vi "main--pop up example.vi"() -> ()   [LabVIEW 2021]
doc: "Example for showing different pop-up types"
uses:
  Graphics.ctl
  Popup/message info--typedef.ctl
  Standard/Two Button/Two Button.lvclass
  Pop-Up.lvlib
  Theme/Theme.lvclass
  Standard/Timeout/Timeout.lvclass
  Standard/One Button/One Button.lvclass
  Standard/Input (DBL)/Input (DBL).lvclass
  Custom/Custom - One Button/Custom - One Button.lvclass
  Popup/Popup.lvclass
  user32.dll
panel:
  in  "close":bool
  out "header":bool caption="Boolean"
  out "Value":dbl
  in  "time (seconds)":dbl=2.0
  out "Choice":bool
  in  "two-button":bool
  in  "timeout":bool
  in  "custom":bool
  in  "one-button":bool
  in  "load":bool
  in  "input-dbl":bool
  # "Run this VI to see calling a few different types of Pop-Ups\n->Uses Standard Images for most (change on block diagram to see other options)"
  # "temporarily applies a new \ntheme"
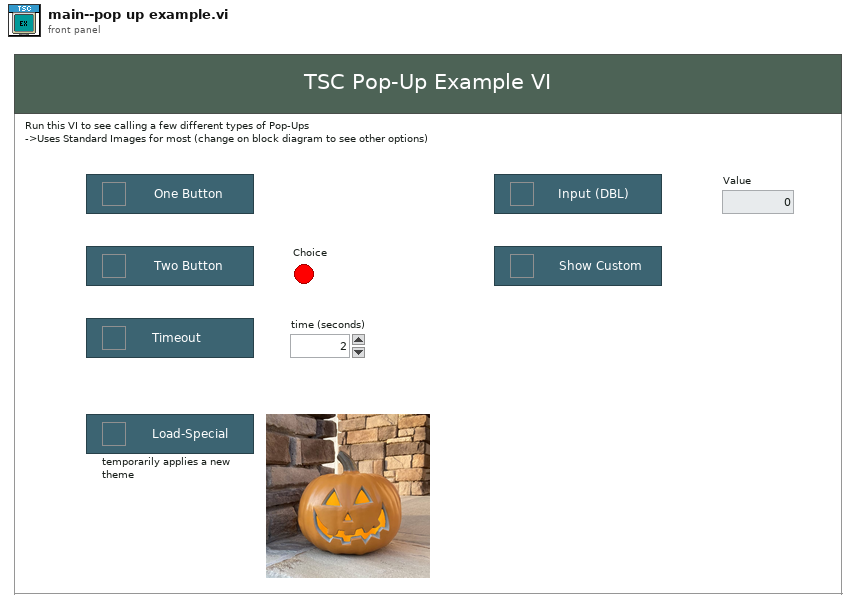
[diagram p1: front panel]
types:
  T1 = typedef "Pop-Up.lvlib/Graphics.ctl" = string
  T2 = typedef "Pop-Up.lvlib/Popup.lvclass/message info--typedef.ctl" = cluster{"Message Height":i32, "Message Width":i32, "Message Location":enum16{"Top", "Bottom", "Right", "Left"}}
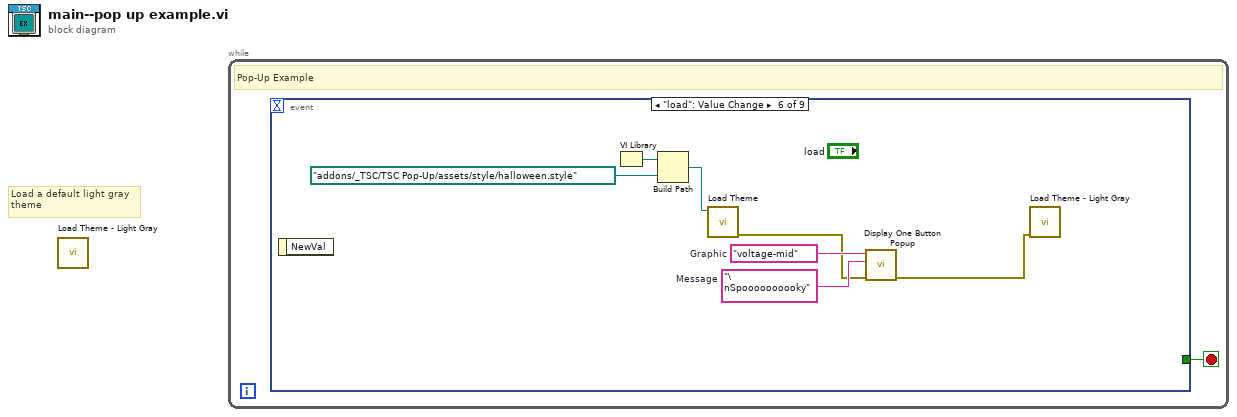
[diagram p0: block diagram]
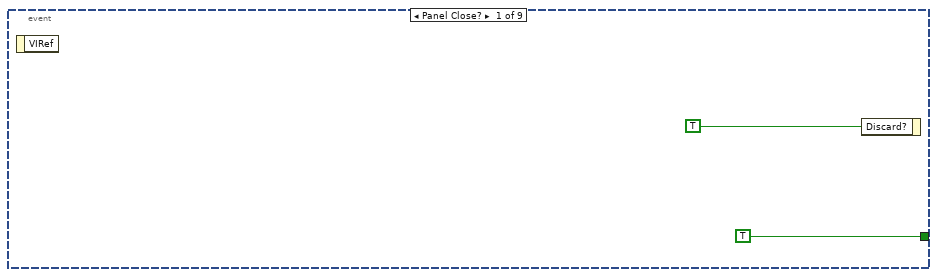
[diagram p2: hidden frame]
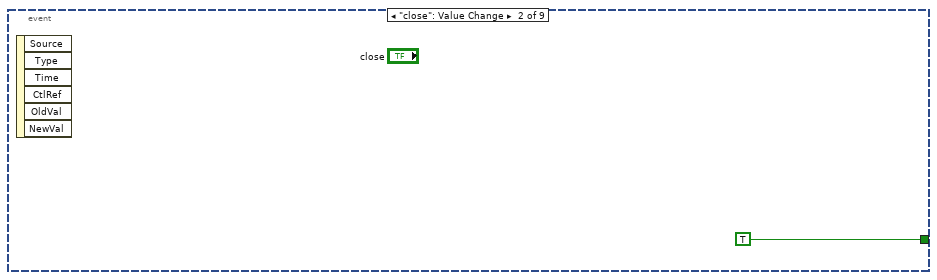
[diagram p3: hidden frame]
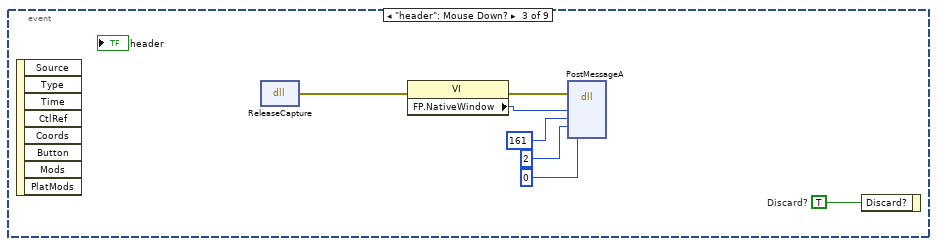
[diagram p4: hidden frame]
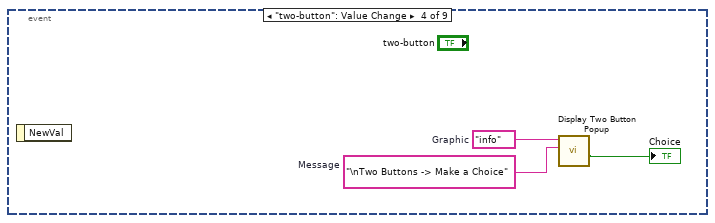
[diagram p5: hidden frame]
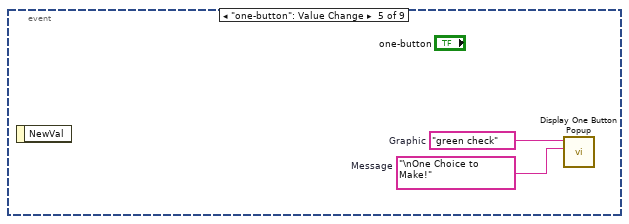
[diagram p6: hidden frame]
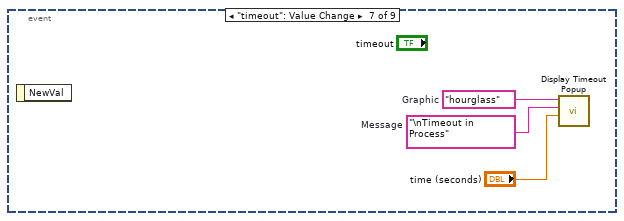
[diagram p7: hidden frame]
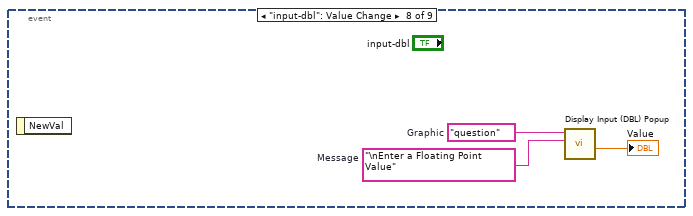
[diagram p8: hidden frame]
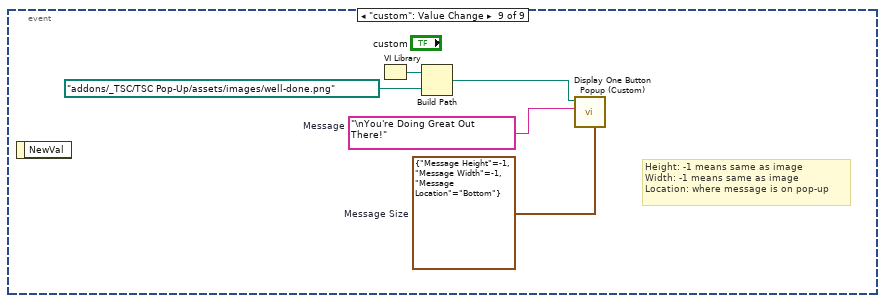
[diagram p9: hidden frame]
diagram:
  # "Load a default light gray\ntheme"
  n1 = call "Load Theme - Light Gray.vi"() -> ()  [unwired: 10 in, 2 out]
  n2 = while {
    stop <- w1 stop-if-true
    # "Pop-Up Example"
    n3 = event shown="[5] \"load\": Value Change" {
      selector: _ -> [_ _ _ _ _ _ _ _ _]
      dyn-events: _ -> [_ _ _ _ _ _ _ _ _]
      timeout: _ -> [_ _ _ _ _ _ _ _ _]
      tunnel: [TRUE TRUE _ _ _ _ _ _ _] -> w1
      event Panel Close? {
        n4 = event-data() -> ()  [unwired: 1 in, 1 out]
        n5 = event-data("Discard?"=TRUE) -> ()  [unwired: 1 in, 1 out]
      }
      event "close": Value Change {
        n6 = event-data() -> ()  [unwired: 1 in, 6 out]
      }
      event "header": Mouse Down? {
        w11 = TRUE  # Discard?
        n7 = event-data() -> ()  [unwired: 1 in, 8 out]
        n8 = dll-call lib="user32.dll" fn="ReleaseCapture"() -> (error out=w7:errorcluster)  [unwired: 4 in, 1 out]
        n9 = property class="VI"(error in=w7) -> (error out=w6:errorcluster, "FP.NativeWindow"=w5:u64)  [unwired: 1 in, 1 out]
        n10 = dll-call lib="user32.dll" fn="PostMessageA"(error in=w6, "hWnd"=w5, "Msg"=161, "wParam"=2, "lParam"=0) -> ()  [unwired: 7 in, 2 out]
        n11 = event-data("Discard?"=w11) -> ()  [unwired: 1 in, 1 out]
      }
      event "two-button": Value Change {
        w13 = "\nTwo Buttons -> Make a Choice"  # Message
        w14 = T1 "info"  # Graphic
        n12 = event-data() -> ()  [unwired: 1 in, 1 out]
        n13 = call "Display Two Button Popup.vi"("Message"=w13, "Graphic"=w14) -> ("Choice"=→"Choice":bool)  [unwired: 8 in, 1 out]
      }
      event "one-button": Value Change {
        w15 = "\nOne Choice to Make!"  # Message
        w16 = T1 "green check"  # Graphic
        n14 = event-data() -> ()  [unwired: 1 in, 1 out]
        n15 = call "Display One Button Popup.vi"("Message"=w15, "Graphic"=w16) -> ()  [unwired: 9 in, 1 out]
      }
      event "load": Value Change {
        w22 = "\nSpoooooooooky"  # Message
        w23 = T1 "voltage-mid"  # Graphic
        n16 = event-data() -> ()  [unwired: 1 in, 1 out]
        n17 = VI Library() -> (path=w19:path)
        n18 = Build Path(base path=w19, name or relative path=path "addons/_TSC/TSC Pop-Up/assets/style/halloween.style") -> (appended path=w17:path)
        n19 = call "Load Theme.vi"("File Path"=w17) -> ("error out"=w21:errorcluster)  [unwired: 9 in, 1 out]
        n20 = call "Display One Button Popup.vi"("error in"=w21, "Message"=w22, "Graphic"=w23) -> ("error out"=w20:errorcluster)  [unwired: 8 in]
        n21 = call "Load Theme - Light Gray.vi"("error in (no error)"=w20) -> ()  [unwired: 9 in, 2 out]
      }
      event "timeout": Value Change {
        w24 = "\nTimeout in Process"  # Message
        w25 = T1 "hourglass"  # Graphic
        n22 = event-data() -> ()  [unwired: 1 in, 1 out]
        n23 = call "Display Timeout Popup.vi"("Timeout (s)"="time (seconds)", "Message"=w24, "Graphic"=w25) -> ()  [unwired: 7 in, 2 out]
      }
      event "input-dbl": Value Change {
        w28 = "\nEnter a Floating Point Value"  # Message
        w29 = T1 "question"  # Graphic
        n24 = event-data() -> ()  [unwired: 1 in, 1 out]
        n25 = call "Display Input (DBL) Popup.vi"("Message"=w28, "Graphic"=w29) -> ("Input Value"=→"Value":dbl)  [unwired: 8 in, 1 out]
      }
      event "custom": Value Change {
        w33 = T2 {"Message Height"=-1, "Message Width"=-1, "Message Location"=enum."Bottom"}  # Message Size
        w34 = "\nYou're Doing Great Out There!"  # Message
        # "Height: -1 means same as image\nWidth: -1 means same as image\nLocation: where message is on pop-up"
        n26 = event-data() -> ()  [unwired: 1 in, 1 out]
        n27 = VI Library() -> (path=w32:path)
        n28 = Build Path(base path=w32, name or relative path=path "addons/_TSC/TSC Pop-Up/assets/images/well-done.png") -> (appended path=w30:path)
        n29 = call "Display One Button Popup (Custom).vi"("Message Size"=w33, "Message"=w34, "Graphic"=w30) -> ()  [unwired: 8 in, 1 out]
      }
    }
  }
